vi "vi_timer.vi"(1 "reinitialize":bool) -> (0 "ms/i":dbl)   [LabVIEW 2011]
panel:
  out "ms":u32
  out "Iterations":i32
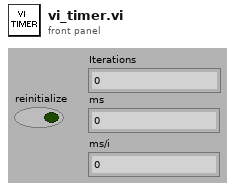
[diagram p1: front panel]
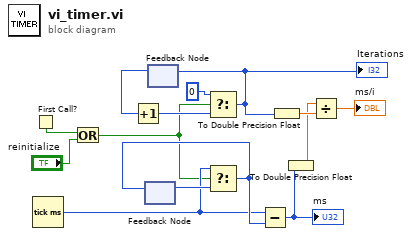
[diagram p0: block diagram]
diagram:
  n1 = First Call?() -> (First Call?: T/F=w7:bool)
  n2 = Tick Count (ms)() -> (millisecond timer value=w11:u32)
  n3 = Or(x=w7, y="reinitialize") -> (x .or. y?=w5:bool)
  n4 = feedback #1() -> (w14:u32)  [unwired: 1 out]
  n5 = feedback #2() -> (w9:i32)  [unwired: 1 out]
  n6 = Increment(x=w9) -> (x+1=w8:i32)
  n7 = Select(t=0, s=w5, f=w8) -> (s? t:f=w3:i32)
  "Iterations" <- w3
  n8 = feedback-in #2(w3) -> ()
  n9 = Select(t=w11, s=w5, f=w14) -> (s? t:f=w12:u32)
  n10 = feedback-in #1(w12) -> ()
  n11 = Subtract(x=w11, y=w12) -> (x-y=w4:u32)
  "ms" <- w4
  n12 = To Double Precision Float(number=w3) -> (double precision float=w2:dbl)
  n13 = To Double Precision Float(number=w4) -> (double precision float=w1:dbl)
  n14 = Divide(x=w1, y=w2) -> (x/y=→"ms/i":dbl)
